vi "Get All Element Labels.vi"(8 "error in":errorcluster, 11 "Class in":refnum<class>) -> (0 "error out":errorcluster, 2 "Labels":string[](array[string]), 3 "Class out":refnum<class>)   [LabVIEW 2023, in "Label-Driven UI.lvlib"]
doc: "VI가 가진 모든 컨트롤과 인디케이터의 라벨들을 얻습니다."
uses:
  Label-Driven UI.lvlib
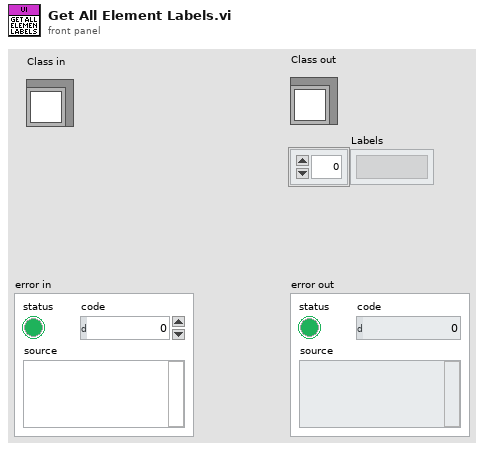
[diagram p1: front panel]
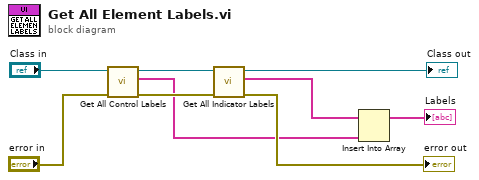
[diagram p0: block diagram]
diagram:
  n1 = call "Get All Control Labels.vi"("error in"="error in", "Class in"="Class in") -> ("error out"=w7:errorcluster, "Labels"=w1:string[], "Class out"=w8:refnum<class>)  [unwired: 7 in]
  n2 = call "Get All Indicator Labels.vi"("error in"=w7, "Class in"=w8) -> ("error out"=→"error out":errorcluster, "Labels"=w3:string[], "Class out"=→"Class out":refnum<class>)  [unwired: 7 in]
  n3 = Insert Into Array(array=w3, new element=w1) -> (→"Labels":string[])  [unwired: 1 in]
